vi "compass.vi"() -> ()   [LabVIEW 2019]
panel:
  out "Gauge 2":dbl(knob) scale=0.0..360.0
  in  "stop":bool
  in  "Slide":u32(slide) max=360 scale=0.0..360.0
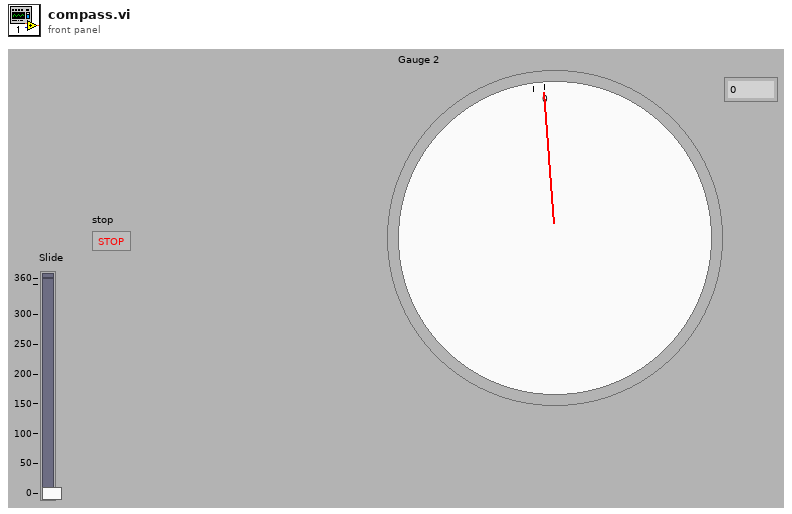
[diagram p1: front panel]
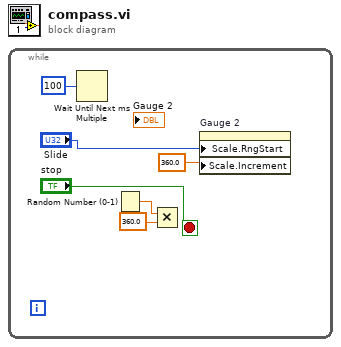
[diagram p0: block diagram]
diagram:
  n1 = while {
    stop <- "stop" stop-if-true
    n2 = Wait Until Next ms Multiple(millisecond multiple=u32 100) -> ()  [unwired: 1 out]
    n3 = Random Number (0-1)() -> (number: 0 to 1=w5:dbl)
    n4 = Multiply(x=w5, y=360.0) -> ()  [unwired: 1 out]
    n5 = property on="Gauge 2" class="Knob (strict)"("Scale.RngStart"="Slide", "Scale.Increment"=360.0 ("Scale.Range:Increment")) -> ()  [unwired: 2 in, 2 out]
  }
